vi "Global procedura abilitata.vi"() -> ()   [LabVIEW 2019]
panel:
  in  "Prova selezionata":i8
  out "Procedura abilitata":bool
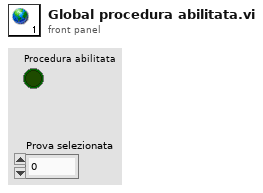
[diagram p1: front panel]
diagram:
